vi "Memory.Pointer.DBL.Write.vi"(8 "error in (no error)":errorcluster, 10 "value":dbl, 11 "DBL Pointer in":refnum<class "Memory.Pointer.DBL.lvclass">) -> (0 "error out":errorcluster, 2 "value out":dbl, 3 "DBL Pointer out":refnum<class "Memory.Pointer.DBL.lvclass">)   [LabVIEW 2016, in "LabVIEW Memory Manager.lvlib" / "Memory.Pointer.DBL.lvclass"]
uses:
  Memory.Pointer.DBL.lvclass
  C:/Users/Ryan/Documents/Git/Sourcetree/LabVIEW-Memory-Manager/Source/Library/Classes/Pointer/Memory.Pointer.Void.lvclass
  Pointer/Memory.Pointer.Void.lvclass/Memory.Pointer.Void.ctl
  Pointer/Memory.Pointer.Void.lvclass
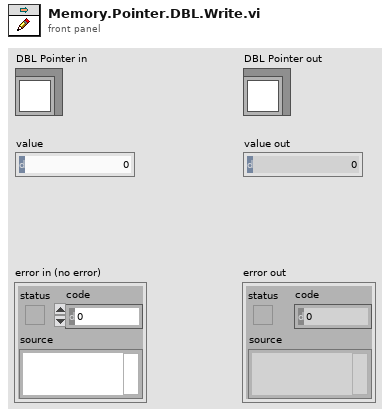
[diagram p1: front panel]
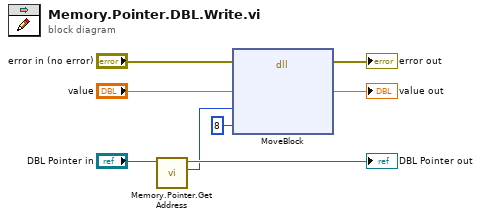
[diagram p0: block diagram]
diagram:
  n1 = call "Memory.Pointer.Get Address.vi"("Pointer in"="DBL Pointer in") -> ("address"=w1:u64, "Pointer out"=→"DBL Pointer out":refnum<class "Memory.Pointer.DBL.lvclass">)  [unwired: 8 in, 1 out]
  n2 = dll-call lib="LabVIEW" fn="MoveBlock"(error in="error in (no error)", "src"="value", "dst"=w1, "size"=u64 8) -> (error out=→"error out":errorcluster, "src"=→"value out":dbl)  [unwired: 5 in, 1 out]
